vi "Configure Arm Layer Real-time Clock.vi"(0 "VISA resource name":refnum<visa-resource-name>, 5 "Date and Time":timestamp, 11 "error in (no error)":errorcluster) -> (4 "VISA resource name out":refnum<visa-resource-name>, 15 "error out":errorcluster)   [LabVIEW 2020, in "Keithley 6517.lvlib"]
doc: "Sets the date and time for the real time clock control source of the Arm Layer (Arm1) of the trigger model.\n\n<B>Note:</B>\n(1)<B>Models 6517A, 6517B:</B> The trigger model consists of 3 layers, the Arm Layer, the Scan Layer (Arm2), and the Measure Layer (Trigger).\n(2)<B>Model 6514:</B> The trigger model consists of 2 layers: Arm Layer & Measure Layer (Trigger).\n\nThis VI is <B>NOT</B> compatible with model <B>6514</B>."
uses:
  <instrlib>/Keithley 6517/Keithley 6517.lvlib
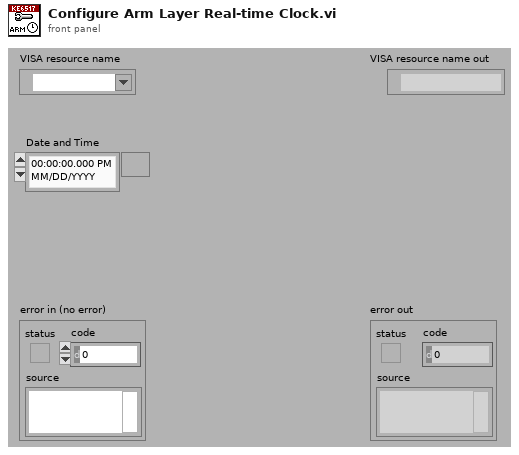
[diagram p1: front panel]
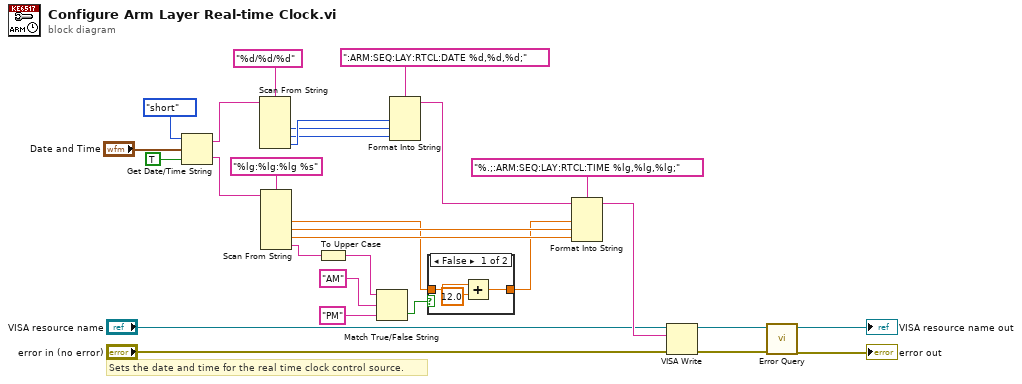
[diagram p0: block diagram]
diagram:
  # "Sets the date and time for the real time clock control source."
  n1 = Get Date/Time String(date format (0)=enum16{"short", "long", "abbreviated"}."short", seconds (now)="Date and Time", want seconds? (F)=TRUE) -> (date string=w16:string, time string=w15:string)
  n2 = Scan From String(format string="%d/%d/%d", input string=w16) -> (output 1=w12:i32, output 2=w11:i32, output 3=w13:i32)  [unwired: 5 in, 3 out]
  n3 = Scan From String(format string="%lg:%lg:%lg %s", input string=w15) -> (output 1=w2:dbl, output 2=w9:dbl, output 3=w8:dbl, output 4=w7:string)  [unwired: 6 in, 3 out]
  n4 = To Upper Case(1:w7) -> (0:w6:string)
  n5 = Match True/False String(2:"PM" ("false string"), 3:"AM" ("true string"), 4:w6) -> (0:w3:bool)  [unwired: 1 out]
  n6 = Format Into String(format string=":ARM:SEQ:LAY:RTCL:DATE %d,%d,%d;", w13, w12, w11) -> (resulting string=w28:string)  [unwired: 2 in, 1 out]
  n7 = case shown="False" w3 {
    tunnel: w2 -> [w31 w33]
    tunnel: [w32 w33] -> w1
    frame False {
      n8 = Add(x=w31, y=12.0) -> (x+y=w32:dbl)
    }
    frame True {
    }
  }
  n9 = Format Into String(format string="%.;:ARM:SEQ:LAY:RTCL:TIME %lg,%lg,%lg;", initial string=w28, w1, w9, w8) -> (resulting string=w26:string)  [unwired: 1 in, 1 out]
  n10 = VISA Write(VISA resource name="VISA resource name", write buffer=w26, error in (no error)="error in (no error)") -> (VISA resource name out=w23:refnum<visa-resource-name>, error out=w22:errorcluster)  [unwired: 1 out]
  n11 = call <instrlib>:"Error Query.vi"("error in (no error)"=w22, "VISA resource name"=w23) -> ("error out"=→"error out":errorcluster, "VISA resource name out"=→"VISA resource name out":refnum<visa-resource-name>)  [unwired: 6 in, 2 out]
